vi "Gas Flow.vi"() -> ()   [LabVIEW 2011]
uses:
  GlobalVariables.vi
panel:
  out "DMHy":string="DMHy"
  out "TMAl #2":string="TMAl #2"
  out "TMAl #1":string="TMAl #1"
  out "TMGa #2":string="TMGa #2"
  out "TMGa #1":string="TMGa #1"
  out "TMIn #2":string="TMIn #2"
  out "Spare":string="Spare"
  out "TMIn #1":string="TMIn #1"
  out "CCl4":string="CCl4"
  out "DEZn":string="DEZn"
  in  "19":bool caption="49"
  in  "20":bool caption="49"
  in  "29":bool caption="49"
  in  "53":bool caption="49"
  in  "54":bool caption="49"
  in  "55":bool caption="49"
  in  "77":bool caption="49"
  in  "78":bool caption="49"
  in  "79":bool caption="49"
  in  "80":bool caption="49"
  in  "56":bool caption="49"
  in  "81":bool caption="49"
  in  "84":bool caption="49"
  in  "24":bool caption="49"
  in  "24":bool caption="49"
  in  "Flip 91/92":bool
  in  "MFC 55":dbl
  out "MFC 54":dbl
  in  "MFC 53":dbl
  out "MFC 52":dbl
  in  "Flip 33/34":bool
  in  "Flip 35/36":bool
  in  "Flip 37/38":bool
  in  "Flip 49/50":bool
  in  "Flip 39/40":bool
  in  "Flip 45/46":bool
  in  "Flip 47/48":bool
  in  "Flip 41/42":bool
  in  "Flip 43/44":bool
  in  "MFC 51":dbl
  out "MFC 50":dbl
  in  "23":bool caption="49"
  in  "25":bool caption="49"
  in  "MFC 49":dbl
  out "MFC 48":dbl
  in  "26":bool caption="49"
  in  "76":bool caption="49"
  in  "75":bool caption="49"
  in  "66":bool caption="49"
  in  "65":bool caption="49"
  in  "68":bool caption="49"
  in  "67":bool caption="49"
  in  "70":bool caption="49"
  in  "69":bool caption="49"
  in  "72":bool caption="49"
  in  "71":bool caption="49"
  in  "74":bool caption="49"
  in  "73":bool caption="49"
  in  "38":bool caption="49"
  in  "37":bool caption="49"
  in  "50":bool caption="49"
  in  "49":bool
  in  "52":bool caption="49"
  in  "51":bool caption="49"
  in  "36":bool caption="49"
  in  "35":bool caption="49"
  in  "34":bool caption="49"
  in  "33":bool caption="49"
  in  "MFC ? 70":dbl
  in  "MFC ? 68":dbl
  in  "MFC ? 66":dbl
  in  "MFC ? 64":dbl
  in  "MFC ? 62":dbl
  in  "MFC ? 52":dbl
  in  "MFC ? 50":dbl
  in  "MFC ? 48":dbl
  in  "MFC 07":dbl
  in  "MFC ? 44":dbl
  in  "MFC ? 42":dbl
  in  "MFC ? 40":dbl
  in  "MFC ? 38":dbl
  in  "MFC ? 36":dbl
  in  "MFC ? 34":dbl
  in  "MFC ? 32":dbl
  in  "MFC ? 30":dbl
  in  "MFC ? 28":dbl
  in  "MFC ? 26":dbl
  in  "MFC ? 24":dbl
  in  "MFC ? 22":dbl
  in  "MFC ? 20":dbl
  out "MFC ? 71":dbl
  out "MFC ? 69":dbl
  out "MFC ? 67":dbl
  out "MFC ? 65":dbl
  out "MFC ? 63":dbl
  in  "MFC ? 18":dbl
  in  "MFC ? 16":dbl
  in  "MFC 47":dbl
  in  "PC 11":dbl
  in  "MFC 02":dbl
  in  "MFC 46":dbl
  in  "MFC10":dbl
  in  "MFC 45":dbl
  in  "MFC 44":dbl
  in  "MFC 01":dbl
  out "MFC ? 53":dbl
  out "MFC ? 51":dbl
  out "MFC ? 49":dbl
  out "MFC 07":dbl
  out "MFC ? 45":dbl
  out "MFC ? 43":dbl
  out "MFC ? 41":dbl
  out "MFC ? 39":dbl
  out "MFC ? 37":dbl
  out "MFC ? 35":dbl
  out "MFC ? 33":dbl
  out "MFC ? 31":dbl
  out "MFC ? 29":dbl
  out "MFC ? 27":dbl
  out "MFC ? 25":dbl
  out "MFC ? 23":dbl
  out "MFC ? 21":dbl
  out "MFC ? 19":dbl
  out "MFC ? 17":dbl
  out "MFC 47":dbl
  out "PC 11":dbl
  out "MFC 02":dbl
  out "MFC 46":dbl
  out "MFC10":dbl
  out "MFC 45":dbl
  out "MFC 44":dbl
  out "MFC 01":dbl
  in  "07":bool caption="49"
  in  "08":bool caption="49"
  in  "08":bool caption="49"
  in  "17":bool caption="49"
  in  "18":bool caption="49"
  in  "18":bool caption="49"
  in  "64":bool caption="49"
  in  "15":bool caption="49"
  in  "16":bool caption="49"
  in  "16":bool caption="49"
  in  "63":bool caption="49"
  in  "13":bool caption="49"
  in  "14":bool caption="49"
  in  "14":bool caption="49"
  in  "62":bool caption="49"
  in  "11":bool caption="49"
  in  "12":bool caption="49"
  in  "12":bool caption="49"
  in  "22":bool caption="49"
  in  "21":bool caption="49"
  in  "22":bool caption="49"
  in  "61":bool caption="49"
  in  "09":bool caption="49"
  in  "57":bool caption="49"
  in  "05":bool caption="49"
  in  "10":bool caption="49"
  in  "10":bool caption="49"
  in  "58":bool caption="49"
  in  "58":bool caption="49"
  in  "06":bool caption="49"
  in  "06":bool caption="49"
  in  "90":bool caption="49"
  in  "03":bool caption="49"
  in  "04":bool caption="49"
  in  "04":bool caption="49"
  in  "01":bool caption="49"
  in  "02":bool caption="49"
  in  "02":bool caption="49"
  in  "59":bool caption="49"
  in  "27":bool caption="49"
  in  "30":bool caption="49"
  in  "94":bool caption="49"
  in  "93":bool caption="49"
  in  "?":bool caption="49"
  in  "28":bool caption="49"
  in  "31":bool caption="49"
  in  "95":bool caption="49"
  in  "96":bool caption="49"
  in  "90":bool caption="49"
  in  "92":bool caption="49"
  in  "91":bool caption="49"
  in  "86":bool caption="49"
  in  "85":bool caption="49"
  in  "48":bool caption="49"
  in  "47":bool caption="49"
  in  "46":bool caption="49"
  in  "45":bool caption="49"
  in  "44":bool caption="49"
  in  "43":bool caption="49"
  in  "42":bool caption="49"
  in  "41":bool caption="49"
  in  "40":bool caption="49"
  in  "39":bool caption="49"
  in  "CloseVi?":bool
  in  "Close":bool
  # "19"
  # "20"
  # "71/72"
  # "TO EBARA"
  # "Arsine"
  # "32"
  # "AsH3 1-DD VENT"
  # "TO TURBO PUMP"
  # "21"
  # "H2"
  # "33"
  # "23"
  # "69/70"
  # "AsH3 1-DD VENT"
  # "22"
  # "AsH3 2-DD VENT"
  # "AsH3 2-DD VENT"
  # "24"
  # "Si2H6 DD VENT"
  # "34"
  # "67/68"
  # "HYDRIDE GROWTH"
  # "Phosphine"
  # "35"
  # "38"
  # "42"
  # "Si2H6 DD VENT"
  # "HYDRIDE VENT"
  # "?"
  # "36"
  # "TO SHROUD"
  # "39"
  # "TO PURGE"
  # "41"
  # "N2"
  # "41"
  # "57"
  # "TO GLOVE BOX"
  # "28"
  # "ALKYL GROWTH"
  # "ALKYL VENT"
  # "27"
  # "ALKYL DD VENT"
  # "57"
  # "28"
  # "09"
  # "08"
  # "54"
  # "07"
  # "52"
  # "06"
  # "50"
  # "05"
  # "48"
  # "04"
  # "37"
  # "56"
  # "03"
  # "46"
  # "02"
  # "01"
  # "44"
  # "27"
  # "55"
  # "17"
  # "53"
  # "16"
  # "51"
  # "15"
  # "49"
  # "14"
  # "13"
  # "43"
  # "12"
  # "11"
  # "47"
  # "45"
  # "10"
  # "VACUUM"
  # "VENT"
  # "TMAl #2"
  # "DMHy"
  # "TMAl #1"
  # "TMGa #2"
  # "TMGa #1"
  # "TMIn #2"
  # "Spare"
  # "TMIn #1"
  # "CCl4"
  # "DEZn"
  # "07"
  # "01"
  # "03"
  # "04"
  # "09"
  # "52"
  # "12"
  # "44"
  # "13"
  # "53"
  # "45"
  # "05"
  # "46"
  # "37"
  # "16"
  # "10"
  # "48"
  # "02"
  # "56"
  # "08"
  # "06"
  # "49"
  # "11"
  # "43"
  # "54"
  # "50"
  # "14"
  # "47"
  # "55"
  # "51"
  # "17"
  # "15"
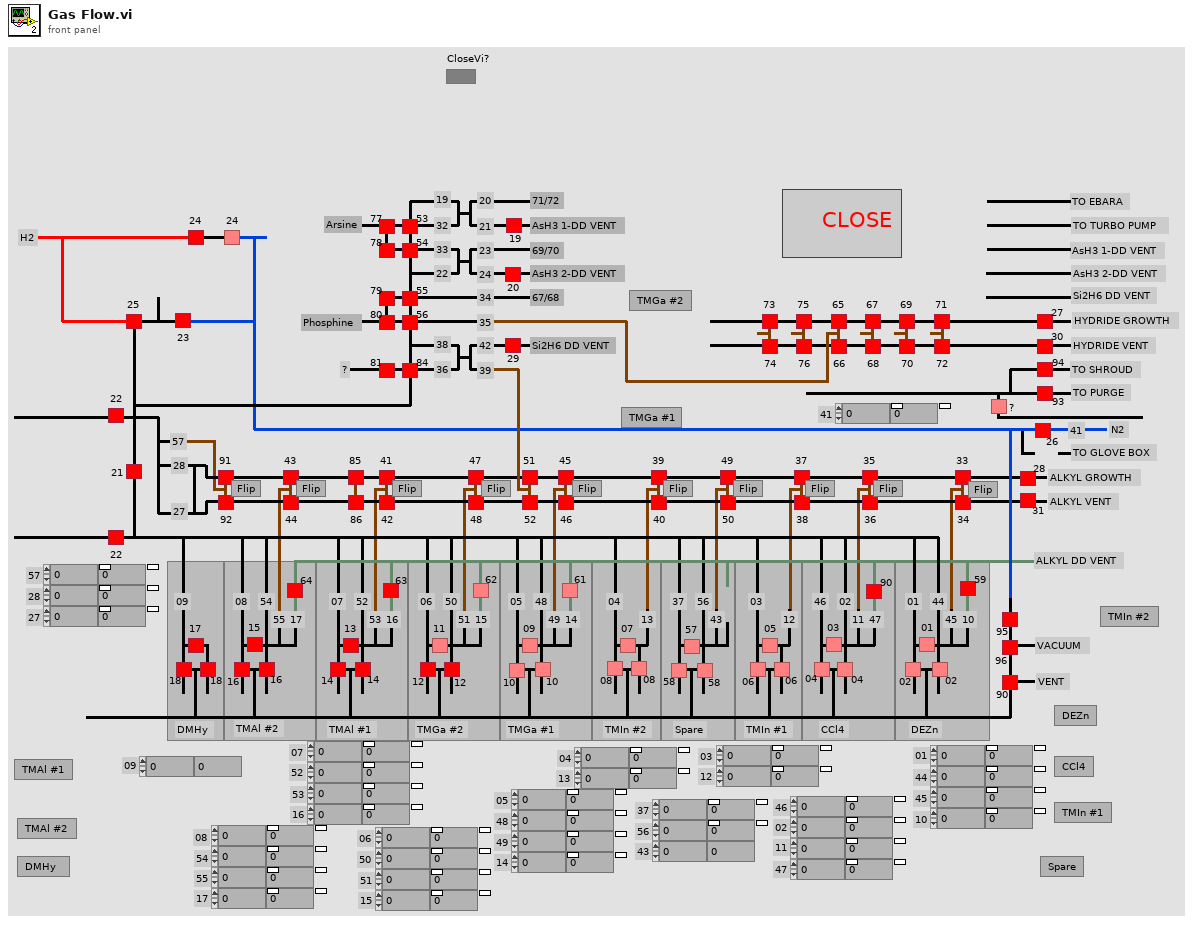
[diagram p1: front panel]
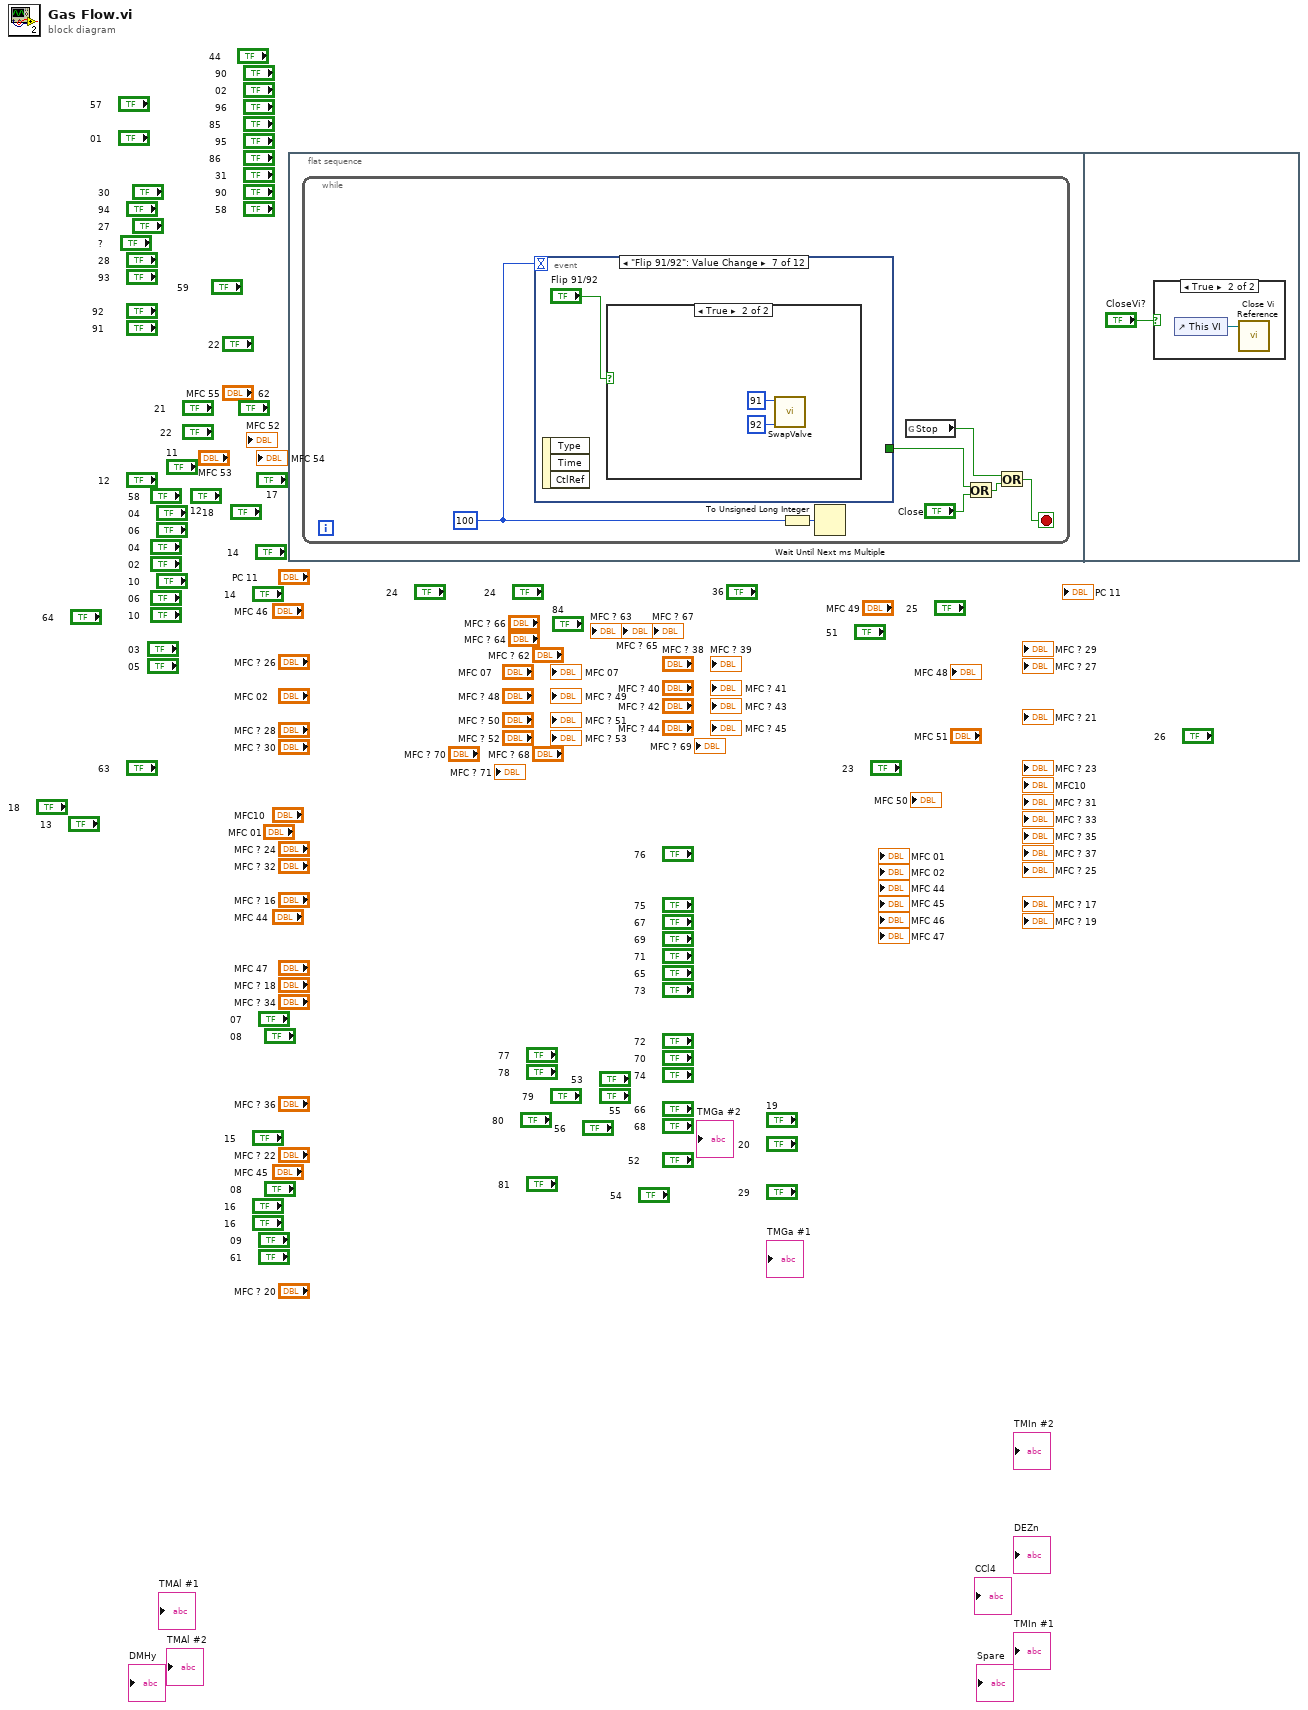
[diagram p0: block diagram]
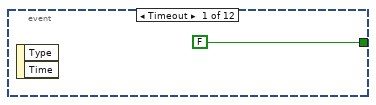
[diagram p2: hidden frame]
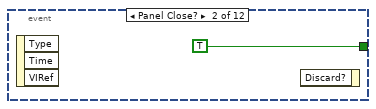
[diagram p3: hidden frame]
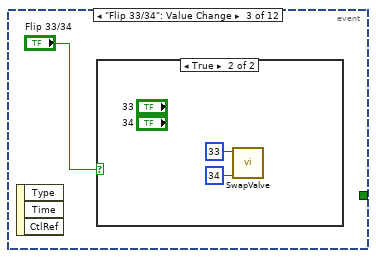
[diagram p4: hidden frame]
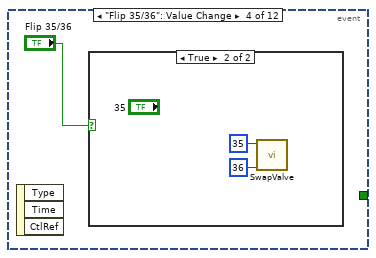
[diagram p6: hidden frame]
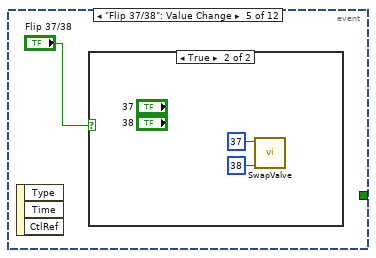
[diagram p8: hidden frame]
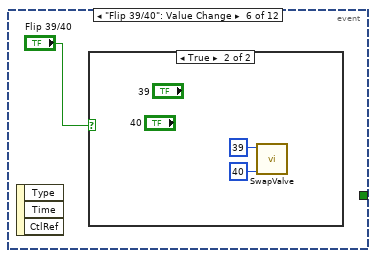
[diagram p10: hidden frame]
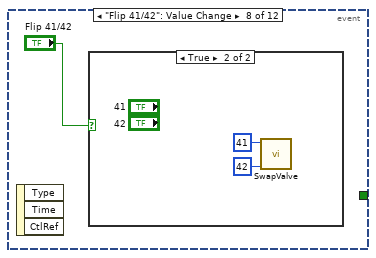
[diagram p13: hidden frame]
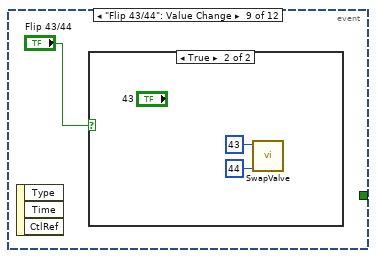
[diagram p15: hidden frame]
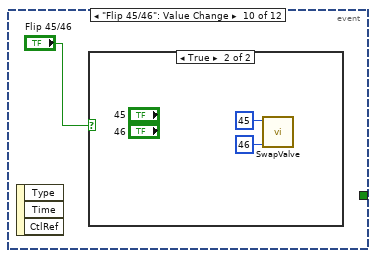
[diagram p17: hidden frame]
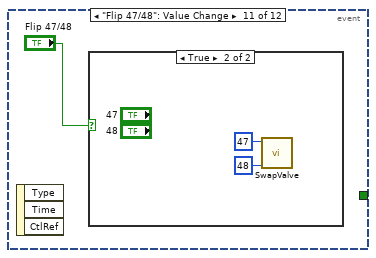
[diagram p19: hidden frame]
diagram:
  n1 = flat-sequence {
    frame #0 {
      n2 = while {
        stop <- w1 stop-if-true
        w2 = 100
        n3 = event shown="[6] \"Flip 91/92\": Value Change" {
          selector: _ -> [_ _ _ _ _ _ _ _ _ _ _ _]
          dyn-events: _ -> [_ _ _ _ _ _ _ _ _ _ _ _]
          timeout: w2 -> [_ _ _ _ _ _ _ _ _ _ _ _]
          tunnel: [FALSE ("y") TRUE ("y") _ _ _ _ _ _ _ _ _ _] -> w4
          event Timeout {
            n4 = event-data() -> ()  [unwired: 1 in, 2 out]
          }
          event Panel Close? {
            n5 = event-data() -> ()  [unwired: 1 in, 3 out]
            n6 = event-data() -> ()  [unwired: 2 in, 1 out]
          }
          event "Flip 33/34": Value Change {
            n7 = event-data() -> ()  [unwired: 1 in, 3 out]
            n8 = case shown="True" "Flip 33/34" {
              frame False {
              }
              frame True {
                n9 = call "SwapValve.vi"("Valve 2"=34, "Valve 1"=33) -> ()  [unwired: 10 in]
              }
            }
          }
          event "Flip 35/36": Value Change {
            n10 = event-data() -> ()  [unwired: 1 in, 3 out]
            n11 = case shown="True" "Flip 35/36" {
              frame False {
              }
              frame True {
                n12 = call "SwapValve.vi"("Valve 2"=36, "Valve 1"=35) -> ()  [unwired: 10 in]
              }
            }
          }
          event "Flip 37/38": Value Change {
            n13 = event-data() -> ()  [unwired: 1 in, 3 out]
            n14 = case shown="True" "Flip 37/38" {
              frame False {
              }
              frame True {
                n15 = call "SwapValve.vi"("Valve 2"=38, "Valve 1"=37) -> ()  [unwired: 10 in]
              }
            }
          }
          event "Flip 39/40": Value Change {
            n16 = event-data() -> ()  [unwired: 1 in, 3 out]
            n17 = case shown="True" "Flip 39/40" {
              frame False {
              }
              frame True {
                n18 = call "SwapValve.vi"("Valve 2"=40, "Valve 1"=39) -> ()  [unwired: 10 in]
              }
            }
          }
          event "Flip 91/92": Value Change {
            n19 = event-data() -> ()  [unwired: 1 in, 3 out]
            n20 = case shown="True" "Flip 91/92" {
              frame False {
              }
              frame True {
                n21 = call "SwapValve.vi"("Valve 2"=92, "Valve 1"=91) -> ()  [unwired: 10 in]
              }
            }
          }
          event "Flip 41/42": Value Change {
            n22 = event-data() -> ()  [unwired: 1 in, 3 out]
            n23 = case shown="True" "Flip 41/42" {
              frame False {
              }
              frame True {
                n24 = call "SwapValve.vi"("Valve 2"=42, "Valve 1"=41) -> ()  [unwired: 10 in]
              }
            }
          }
          event "Flip 43/44": Value Change {
            n25 = event-data() -> ()  [unwired: 1 in, 3 out]
            n26 = case shown="True" "Flip 43/44" {
              frame False {
              }
              frame True {
                n27 = call "SwapValve.vi"("Valve 2"=44, "Valve 1"=43) -> ()  [unwired: 10 in]
              }
            }
          }
          event "Flip 45/46": Value Change {
            n28 = event-data() -> ()  [unwired: 1 in, 3 out]
            n29 = case shown="True" "Flip 45/46" {
              frame False {
              }
              frame True {
                n30 = call "SwapValve.vi"("Valve 2"=46, "Valve 1"=45) -> ()  [unwired: 10 in]
              }
            }
          }
          event "Flip 47/48": Value Change {
            n31 = event-data() -> ()  [unwired: 1 in, 3 out]
            n32 = case shown="True" "Flip 47/48" {
              frame False {
              }
              frame True {
                n33 = call "SwapValve.vi"("Valve 2"=48, "Valve 1"=47) -> ()  [unwired: 10 in]
              }
            }
          }
          event "Flip 49/50": Value Change {
            n34 = event-data() -> ()  [unwired: 1 in, 3 out]
            n35 = case shown="True" "Flip 49/50" {
              frame False {
              }
              frame True {
                n36 = call "SwapValve.vi"("Valve 2"=50, "Valve 1"=49) -> ()  [unwired: 10 in]
              }
            }
          }
        }
        n37 = To Unsigned Long Integer(number=w2) -> (unsigned 32bit integer=w3:u32)
        n38 = Wait Until Next ms Multiple(millisecond multiple=w3) -> ()  [unwired: 1 out]
        n39 = global read "GlobalVariables.vi" "Stop"() -> (w7:bool)
        n40 = Or(x=w4, y="Close") -> (x .or. y?=w6:bool)
        n41 = Or(x=w7, y=w6) -> (x .or. y?=w1:bool)
      }
    }
    frame #1 {
      n42 = case shown="True" "CloseVi?" {
        frame False {
        }
        frame True {
          n43 = control-ref of="This VI"() -> (w41:refnum<vi>)
          n44 = call "Close Vi Reference.vi"("reference"=w41) -> ()  [unwired: 9 in, 2 out]
        }
      }
    }
  }
